vi "Update Connection.vi"(8 "error in (no error)":errorcluster, 10 "TCP Data before update":T1, 11 "TCP Data after update":T1) -> (0 "error out":errorcluster, 3 "TCP Data after update out":T1)   [LabVIEW 2016, in "TCP.lvlib"]
uses:
  TCP.lvlib
  TypeDefs/TCP Data.ctl
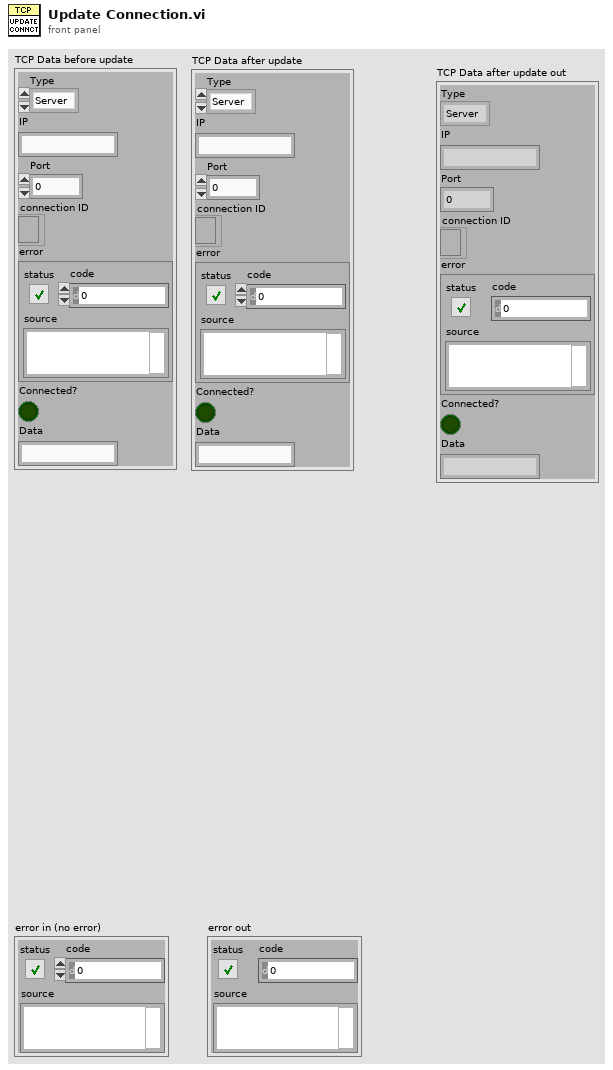
[diagram p1: front panel]
types:
  T1 = typedef "TCP.lvlib/TCP Data.ctl" = cluster{"Type":enum16{"Server", "Client"}, "IP":string, "Port":u16, "connection ID":refnum<k5>, "error":errorcluster, "Connected?":bool, "Data":string}
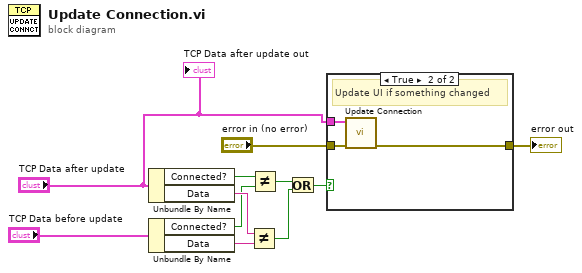
[diagram p0: block diagram]
diagram:
  n1 = Unbundle By Name("TCP Data after update") -> ("Connected?"=w3:bool, "Data"=w5:string)
  n2 = Unbundle By Name("TCP Data before update") -> ("Connected?"=w4:bool, "Data"=w6:string)
  n3 = Not Equal?(x=w5, y=w6) -> (x != y?=w8:bool)
  n4 = Not Equal?(x=w3, y=w4) -> (x != y?=w7:bool)
  n5 = Or(x=w7, y=w8) -> (x .or. y?=w9:bool)
  n6 = case shown="True" w9 {
    tunnel: "error in (no error)" -> [w12 w14]
    tunnel: [w12 w15] -> w11
    tunnel: "TCP Data after update" -> [_ w13]
    frame False {
    }
    frame True {
      # "Update UI if something changed"
      n7 = call "Update Connection.vi"("error in"=w14, "TCP Data"=w13) -> ("error out"=w15:errorcluster)  [unwired: 9 in]
    }
  }
  "error out" <- w11
  "TCP Data after update out" <- "TCP Data after update"
